vi "TCP-Write (2D DBL).vi"(0 "connection ID":refnum<k5>, 5 "data string":dbl[][](array[numeric]), 9 "timeout (ms)":i32=5000, 11 "error in (no error)":errorcluster) -> (4 "connection ID out":refnum<k5>, 8 "bytes written":i32, 15 "error out":errorcluster)   [LabVIEW 2015]
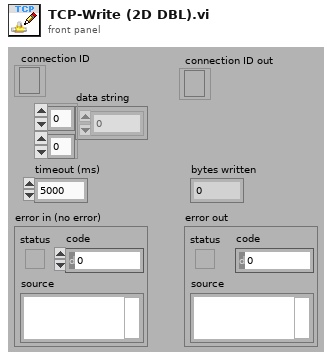
[diagram p1: front panel]
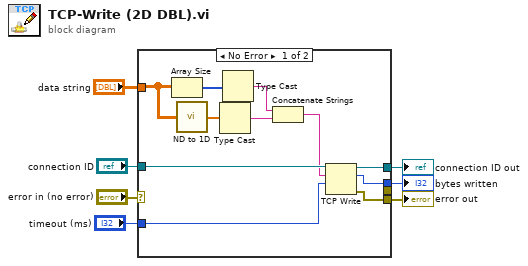
[diagram p0: block diagram]
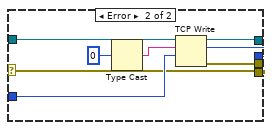
[diagram p2: hidden frame]
diagram:
  n1 = case shown="No Error" "error in (no error)" {
    selector: "error in (no error)" -> [_ w20]
    tunnel: [w8 w20] -> w1
    tunnel: [w18 w25] -> w7
    tunnel: "connection ID" -> [w14 w26]
    tunnel: "timeout (ms)" -> [w16 w23]
    tunnel: [w15 w24] -> w4
    tunnel: "data string" -> [w11 _]
    tunnel: [_ w19] -> _
    frame No Error {
      n2 = Array Size(array=w11) -> (size(s)=w12:i32[])
      n3 = call "ND to 1D.vi"("ND Array"=w11) -> ("1D Array"=w10:dbl[])
      n4 = Type Cast(x=w10) -> (*(type *) &x=w17:string)  [unwired: 1 in]
      n5 = Type Cast(x=w12) -> (*(type *) &x=w9:string)  [unwired: 1 in]
      n6 = Concatenate Strings(w9, w17) -> (w13:string)
      n7 = TCP Write(connection ID=w14, data in=w13, 9:w16) -> (connection ID out=w18:refnum<k5>, bytes written=w15:i32, error out=w8:errorcluster)  [unwired: 1 in]
    }
    frame Error {
      n8 = Type Cast(x=0 ("bytes written")) -> (*(type *) &x=w22:string)  [unwired: 1 in]
      n9 = TCP Write(connection ID=w26, data in=w22, 9:w23) -> (connection ID out=w25:refnum<k5>, bytes written=w24:i32, error out=w19:errorcluster)  [unwired: 1 in]
    }
  }
  "error out" <- w1
  "bytes written" <- w4
  "connection ID out" <- w7
